vi "Iniv_save_VI.vi"(8 "error in (no error)":errorcluster, 11 "Control-Client in":refnum<class "Control-Client.lvclass">) -> (0 "error out":errorcluster, 3 "Control-Client out":refnum<class "Control-Client.lvclass">)   [LabVIEW 2015, in "Control-Client.lvclass"]
uses:
  Control-Client.lvclass
  dependecies/ControlsVIs/Clusters-def/Message types.ctl
  Message/Message.lvclass/Message.ctl
  Control-Client.lvclass/Control-Client.ctl
  Message/Message.lvclass
  GeneralFunctionality/GeneralFunctionality.lvclass
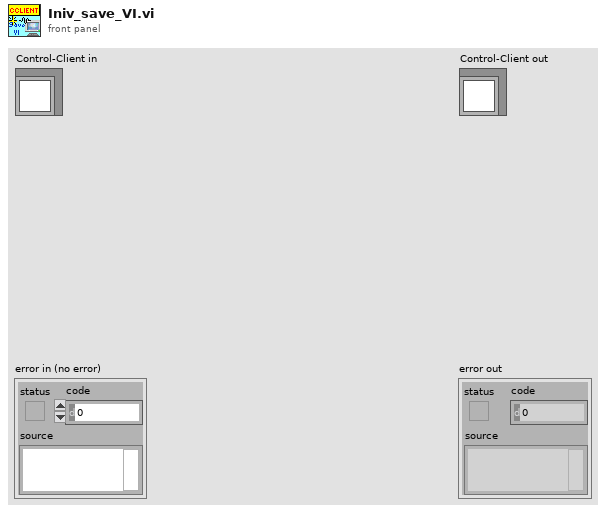
[diagram p1: front panel]
types:
  T1 = typedef "Message types.ctl" = string
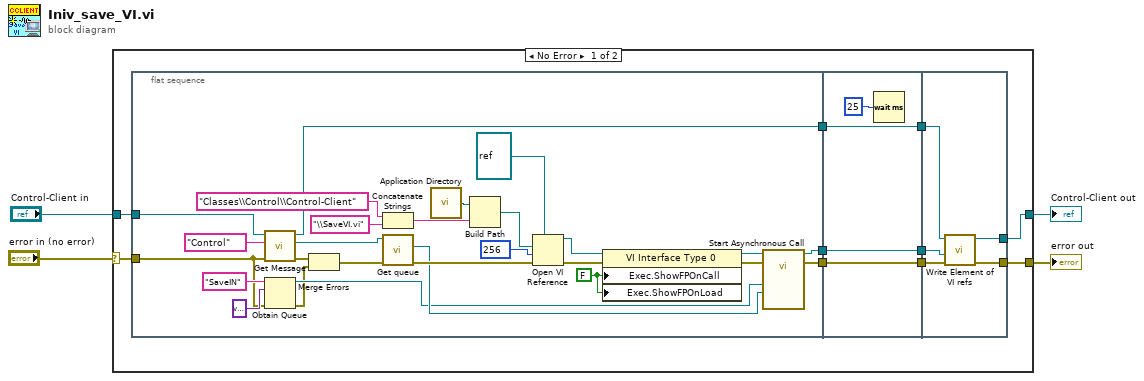
[diagram p0: block diagram]
diagram:
  n1 = case shown="No Error" "error in (no error)" {
    selector: "error in (no error)" -> [w7 w51]
    tunnel: [w10 w52] -> w2
    tunnel: "Control-Client in" -> [w8 w52]
    tunnel: [w9 w51] -> w1
    frame No Error {
      n2 = flat-sequence {
        tunnel: [w41] -> w14
        tunnel: [w30] -> w13
        tunnel: w8 -> [w26]
        tunnel: w7 -> [w18]
        tunnel: [w23] -> w6
        tunnel: w14 -> [w45]
        tunnel: [w45] -> w12
        tunnel: w13 -> [w44]
        tunnel: [w44] -> w11
        tunnel: w6 -> [w42]
        tunnel: [w42] -> w5
        tunnel: w12 -> [w48]
        tunnel: w11 -> [w49]
        tunnel: [w50] -> w10
        tunnel: [w47] -> w9
        tunnel: w5 -> [w46]
        frame #0 {
          w32 = FALSE ("Exécution:Afficher la face-avant à l'appel")
          n3 = call "Get Message.vi"("error in (no error)"=w18, "Message type"=T1 "Control", "GeneralFunctionality en entrée"=w26) -> ("error out"=w17:errorcluster, "Message.lvclass"=w28:refnum<class "Message.lvclass">, "GeneralFunctionality en sortie"=w23:refnum<class "Control-Client.lvclass">)  [unwired: 6 in]
          n4 = Obtain Queue(name (unnamed)="SaveIN", element data type=variant, error in (no error)=w18) -> (queue out=w19:refnum<queue>, error out=w16:errorcluster)  [unwired: 2 in, 1 out]
          n5 = Merge Errors(w17, w16) -> (w15:errorcluster)
          n6 = Concatenate Strings("Classes\\Control\\Control-Client" ("chaîne"), "\\SaveVI.vi" ("chaîne")) -> (w38:string)
          n7 = call "Get queue.vi"("error in (no error)"=w15, "Message in"=w28) -> ("error out"=w25:errorcluster, "queue"=w20:refnum<queue>)  [unwired: 7 in, 1 out]
          n8 = call <vilib>:"Application Directory.vi"() -> ("Application Directory"=w36:path)
          n9 = Build Path(base path=w36, name or relative path=w38) -> (appended path=w35:path)
          n10 = Open VI Reference(type specifier VI Refnum (for type only)=refnum<vi> refnum ("spécificateur de type du refnum de VI (pour type seulement)"), vi path=w35, options=256, error in (no error)=w25) -> (vi reference=w34:refnum<vi>, error out=w33:errorcluster)  [unwired: 2 in]
          n11 = property class="VI Interface Type 0"(reference=w34, error in=w33, "Exec.ShowFPOnCall"=w32, "Exec.ShowFPOnLoad"=w32) -> (reference out=w27:refnum<vi>, error out=w24:errorcluster)
          n12 = call-by-ref "Start Asynchronous Call"(reference=w27, error in=w24, "queueOUT"=w20, "queueIN"=w19) -> (reference out=w30:refnum<vi>, error out=w41:errorcluster)  [unwired: 10 in]
        }
        frame #1 {
          n13 = Wait (ms)(milliseconds to wait=u32 25) -> ()  [unwired: 1 out]
        }
        frame #2 {
          n14 = call "Write Element of VI refs.vi"("error in (no error)"=w48, "vi reference"=w49, "Control-Client in"=w46) -> ("error out"=w47:errorcluster, "Control-Client out"=w50:refnum<class "Control-Client.lvclass">)  [unwired: 7 in]
        }
      }
    }
    frame Error {
    }
  }
  "error out" <- w1
  "Control-Client out" <- w2
